vi "LVCompareGitAdapter.vi"   [LabVIEW 2017]
uses:
  <vilib>/Utility/config.llb/Read Key (String).vi
  <vilib>/Utility/config.llb/NI_LVConfig.lvlib
types:
  T1 = enum32{"Invalid", "Standard", "Closed", "Hidden", "Minimized", "Maximized"}
  T2 = typedef "NI_LVConfig.lvlib/Config Data RefNum.ctl" = refnum<k1>
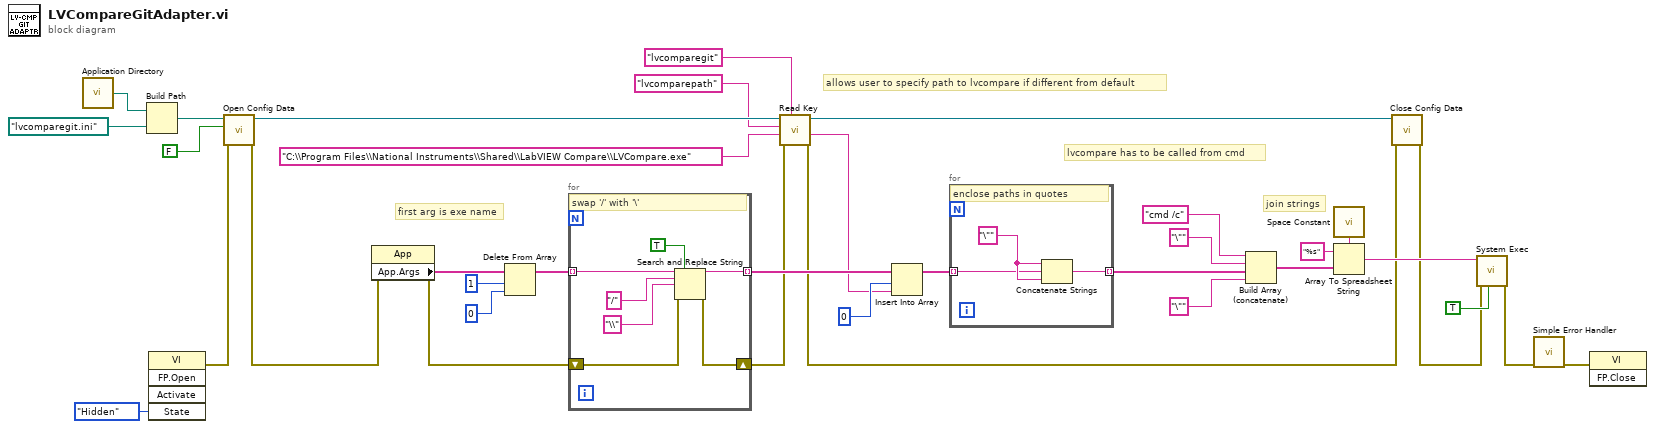
[diagram p0: block diagram]
diagram:
  # "allows user to specify path to lvcompare if different from default"
  # "join strings"
  # "first arg is exe name"
  # "lvcompare has to be called from cmd"
  n1 = call <vilib>:"Application Directory.vi"() -> ("Application Directory"=w10:path)
  n2 = Build Path(base path=w10, name or relative path=path "lvcomparegit.ini" ("configuration file path")) -> (appended path=w8:path)
  n3 = invoke class="VI" method="FP.Open"("State"=T1."Hidden") -> (error out=w6:errorcluster)  [unwired: 4 in, 4 out]
  n4 = call <vilib>:"Open Config Data.vi"("error in (no error)"=w6, "create file if necessary (T)"=FALSE, "configuration file path"=w8) -> ("error out"=w13:errorcluster, "refnum"=w17:T2)  [unwired: 6 in, 1 out]
  n5 = property class="App"(error in=w13) -> (error out=w18:errorcluster, "App.Args"=w33:string[])  [unwired: 1 in, 1 out]
  n6 = Delete From Array(array=w33, length=1, index=0) -> (array with subset deleted=w32:string[])  [unwired: 1 out]
  n7 = for {
    tunnel: w32 -> [w39] mode=indexing
    tunnel: [w36] -> w25 mode=indexing
    shift-right: [w37] -> w5
    shift-left: w18 -> [w38]
    # "swap '/' with '\\'"
    n8 = Search and Replace String(replace all?=TRUE ("ignore case? (F)"), input string=w39, search string="/", replace string="\\" ("replace string (\"\")"), error in=w38) -> (result string=w36:string, error out=w37:errorcluster)  [unwired: 3 in, 2 out]
  }
  n9 = call-poly <vilib>:"Read Key.vi"("section"="lvcomparegit", "error in (no error)"=w5, "default value"="C:\\Program Files\\National Instruments\\Shared\\LabVIEW Compare\\LVCompare.exe" ("result string"), "key"="lvcomparepath", "refnum"=w17) -> ("error out"=w4:errorcluster, "value"=w14:string, "refnum out"=w12:T2)  [unwired: 3 in, 1 out]
  n10 = Insert Into Array(array=w25, index=0, new element=w14) -> (w24:string[])
  n11 = for {
    tunnel: w24 -> [w44] mode=indexing
    tunnel: [w43] -> w27 mode=indexing
    w45 = "\"" ("result string")
    # "enclose paths in quotes"
    n12 = Concatenate Strings(w45, w44, w45) -> (w43:string)
  }
  n13 = Build Array (concatenate)("cmd /c" ("result string"), "\"" ("result string"), w27, "\"" ("result string")) -> (w26:string[])
  n14 = call <vilib>:"Space Constant.vi"() -> ("String"=w34:string)
  n15 = Array To Spreadsheet String(delimiter (Tab)=w34, array=w26, 3:"%s" ("format string")) -> (spreadsheet string=w29:string)
  n16 = call <vilib>:"Close Config Data.vi"("error in (no error)"=w4, "refnum"=w12) -> ("error out"=w3:errorcluster)  [unwired: 8 in, 1 out]
  n17 = call <vilib>:"System Exec.vi"("run minimized? (F)"=TRUE, "error in (no error)"=w3, "command line"=w29) -> ("error out"=w2:errorcluster)  [unwired: 5 in, 3 out]
  n18 = call <vilib>:"Simple Error Handler.vi"("error in (no error)"=w2) -> ("error out"=w1:errorcluster)  [unwired: 4 in, 4 out]
  n19 = invoke class="VI" method="FP.Close"(error in=w1) -> ()  [unwired: 2 in, 3 out]
